vi "SendProgramClose.vi"(8 "error in (no error)":errorcluster, 11 "Queue in":refnum<queue>) -> ()   [LabVIEW 2014, in "ProgramClose.lvclass"]
uses:
  ProgramClose.lvclass
  AbstractionMessage/AbstractionMessage.lvclass
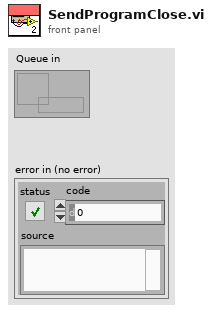
[diagram p1: front panel]
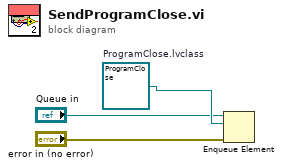
[diagram p0: block diagram]
diagram:
  w3 = refnum<class "ProgramClose.lvclass"> refnum  # ProgramClose.lvclass
  n1 = Enqueue Element(queue="Queue in", element=w3, error in (no error)="error in (no error)") -> ()  [unwired: 1 in, 3 out]
